vi "Write Data (Byte Array).vi"(8 "error in (no error)":errorcluster, 10 "Write Buffer":u8[](array[numeric]) format="%x", 11 "Handle":u64) -> (0 "error out":errorcluster, 2 "Bytes Written":u32, 3 "Handle out":u64)   [LabVIEW 2019, in "D2XX-lv.lvlib"]
doc: "Write byte array data to the open device."
uses:
  D2XX-lv.lvlib
  <instrlib>/_D2XX/D2XX/D2XX.lvlib
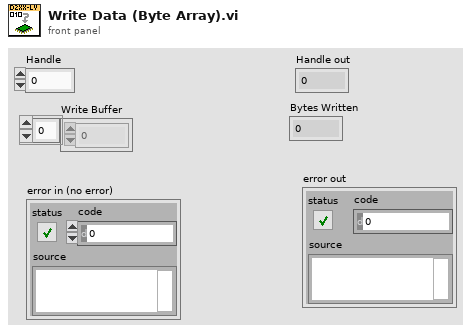
[diagram p1: front panel]
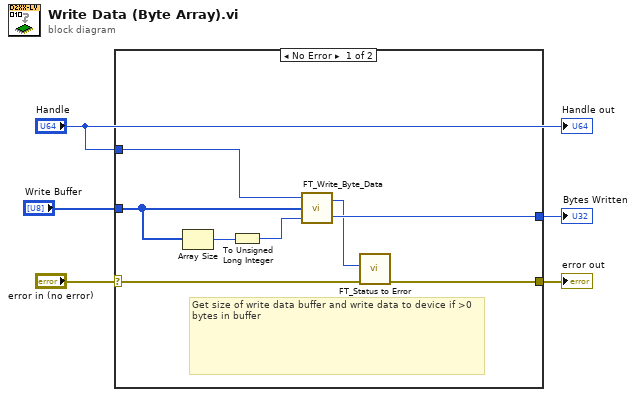
[diagram p0: block diagram]
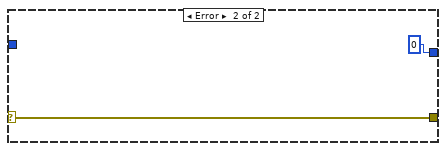
[diagram p2: hidden frame]
diagram:
  n1 = case shown="No Error" "error in (no error)" {
    selector: "error in (no error)" -> [w13 w15]
    tunnel: [w12 w15] -> w4
    tunnel: "Handle" -> [w7 _]
    tunnel: [w9 u32 0 ("Bytes Written")] -> w3
    tunnel: "Write Buffer" -> [w6 _]
    frame No Error {
      # "Get size of write data buffer and write data to device if >0 bytes in buffer"
      n2 = Array Size(array=w6) -> (size(s)=w11:i32)
      n3 = To Unsigned Long Integer(number=w11) -> (unsigned 32bit integer=w10:u32)
      n4 = call <instrlib>:"FT_Write_Byte_Data.vi"("Bytes To Write"=w10, "Buffer"=w6, "Handle"=w7) -> ("Bytes Written"=w9:u32, "FT_Status"=w8:u32)
      n5 = call "FT_Status to Error.vi"("error in (no error)"=w13, "FT_Status"=w8) -> ("error out"=w12:errorcluster)  [unwired: 9 in]
    }
    frame Error {
    }
  }
  "error out" <- w4
  "Bytes Written" <- w3
  "Handle out" <- "Handle"
